vi "电压采样检测.vi"() -> ()   [LabVIEW 2020]
uses:
  D/Program Files (x86)/National Instruments/LabVIEW 2020/instr.lib/Keithley 24XX/Public/Data/Read (Single Point).vi
  D/Program Files (x86)/National Instruments/LabVIEW 2020/instr.lib/Keithley 24XX/Keithley 24XX.lvlib
panel:
  out "表格控件":string[][](table) caption="电压采样精度检测"
  out "?":bool
  out "电压 3":cluster{"Va":u32, "Vc":u32, "Vd":u32, "Vg":u32}
  out "闭合主正+快充":cluster{"Va":u32, "Vc":u32, "Vd":u32, "Vg":u32}
  in  "VISA resource name":refnum<visa-resource-name>
  out "闭合主正":cluster{"Va":u32, "Vc":u32, "Vd":u32, "Vg":u32}
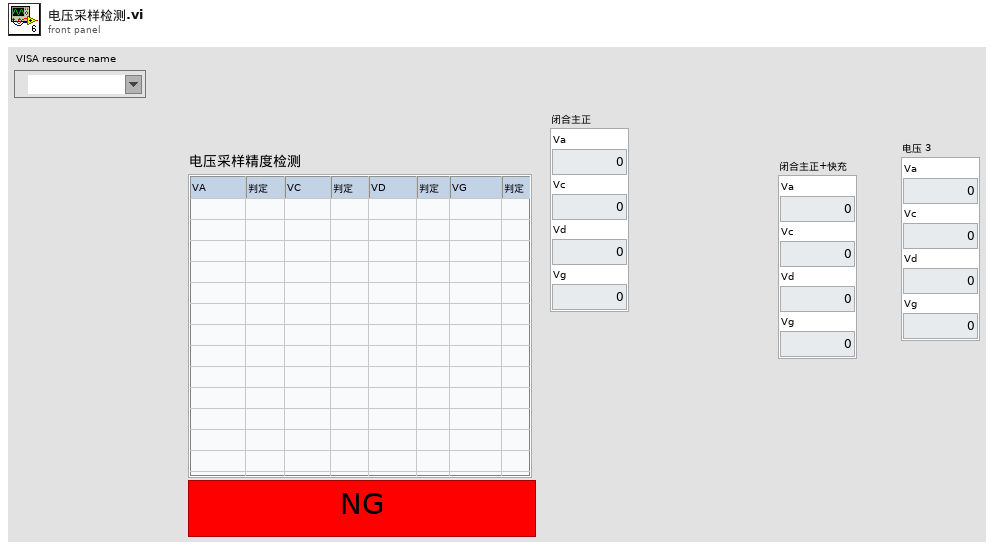
[diagram p1: front panel]
types:
  T1 = cluster{"电压[0]":u32, "电压[1]":u32, "电压[2]":u32, "电压[3]":u32}
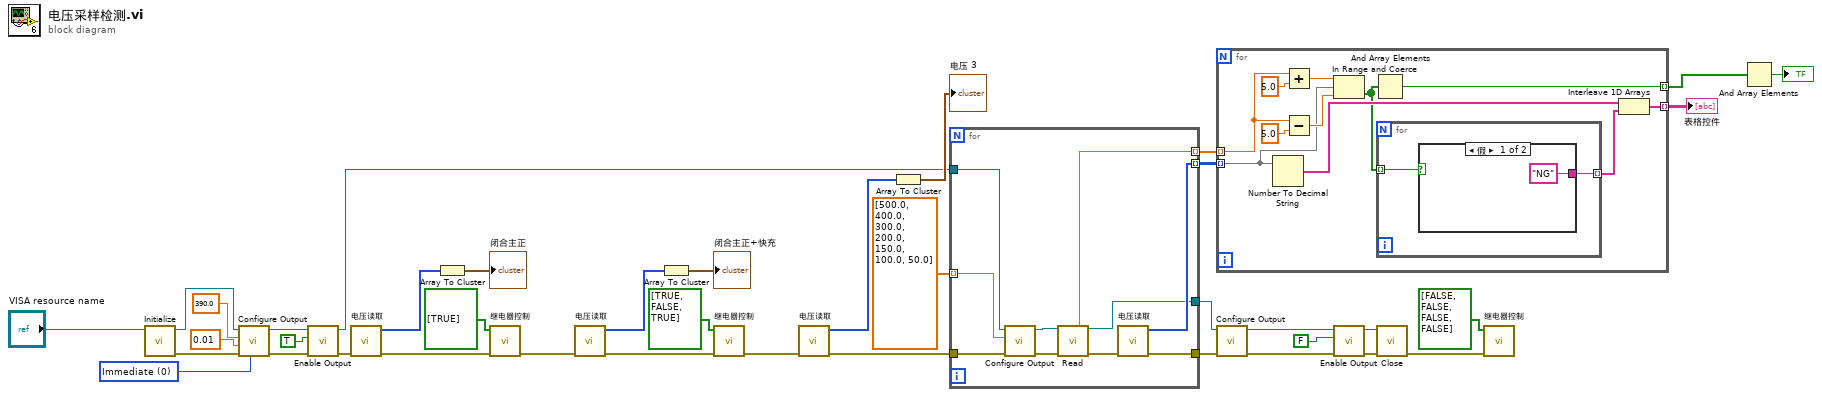
[diagram p0: block diagram]
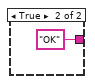
[diagram p2: hidden frame]
diagram:
  w32 = u16 0 items=["Immediate", "Triggered"] ("Output Type  (0: Immediate)")
  n1 = call "Initialize.vi"("VISA resource name"="VISA resource name") -> ("error out"=w33:errorcluster, "VISA resource name out"=w34:refnum<visa-resource-name>)  [unwired: 9 in]
  n2 = call "Configure Output.vi"("Output Type  (0: Immediate)"=w32, "error in (no error)"=w33, "Compliance  Level (0.1)"=0.01, "Output Level (0)"=390.0, "VISA resource name"=w34) -> ("error out"=w31:errorcluster, "VISA resource name out"=w30:refnum<visa-resource-name>)  [unwired: 5 in]
  n3 = call "Enable Output.vi"("error in (no error)"=w31, "Enable Output (T: Enable)"=TRUE, "VISA resource name"=w30) -> ("error out"=w28:errorcluster, "VISA resource name out"=w16:refnum<visa-resource-name>)  [unwired: 7 in]
  n4 = call "电压读取.vi"("error in"=w28) -> ("error out"=w27:errorcluster, "电压"=w39:u32[])  [unwired: 9 in]
  n5 = Array To Cluster(array=w39) -> (cluster=→"闭合主正":T1)
  n6 = call "继电器控制.vi"("error in"=w27, "继电器控制"=bool[] [TRUE]) -> ("error out"=w25:errorcluster)  [unwired: 9 in]
  n7 = call "电压读取.vi"("error in"=w25) -> ("error out"=w22:errorcluster, "电压"=w23:u32[])  [unwired: 9 in]
  n8 = Array To Cluster(array=w23) -> (cluster=→"闭合主正+快充":T1)
  n9 = call "继电器控制.vi"("error in"=w22, "继电器控制"=bool[] [TRUE, FALSE, TRUE]) -> ("error out"=w20:errorcluster)  [unwired: 9 in]
  n10 = call "电压读取.vi"("error in"=w20) -> ("error out"=w6:errorcluster, "电压"=w18:u32[])  [unwired: 9 in]
  n11 = Array To Cluster(array=w18) -> (cluster=→"电压 3":T1)
  n12 = for {
    tunnel: dbl[] [500.0, 400.0, 300.0, 200.0, 150.0, 100.0, 50.0] -> [w49] mode=indexing
    tunnel: w16 -> [w48]
    tunnel: [w47] -> w15
    tunnel: [w41] -> w14
    tunnel: [w46] -> w5 mode=indexing
    tunnel: w6 -> [w45]
    tunnel: [w40] -> w4 mode=indexing
    n13 = call "Configure Output.vi"("error in (no error)"=w45, "Output Level (0)"=w49, "VISA resource name"=w48) -> ("error out"=w44:errorcluster, "VISA resource name out"=w42:refnum<visa-resource-name>)  [unwired: 7 in]
    n14 = call-poly "Read.vi"("VISA resource name"=w42, "error in (no error)"=w44) -> ("Voltage"=w40:sgl, "VISA resource name out"=w41:refnum<visa-resource-name>, "error out"=w43:errorcluster)  [unwired: 7 in, 4 out]
    n15 = call "电压读取.vi"("error in"=w43) -> ("error out"=w47:errorcluster, "电压"=w46:u32[])  [unwired: 9 in]
  }
  n16 = for {
    tunnel: w5 -> [w55] mode=indexing
    tunnel: w4 -> [w58] mode=indexing
    tunnel: [w52] -> w1 mode=indexing
    tunnel: [w50] -> w3 mode=indexing
    n17 = Number To Decimal String(number=w55) -> (decimal integer string=w54:string[])  [unwired: 1 in]
    n18 = Add(x=w58, y=5.0) -> (x+y=w57:dbl)
    n19 = Subtract(x=w58, y=5.0) -> (x-y=w56:dbl)
    n20 = In Range and Coerce(upper limit=w57, x=w55, lower limit=w56) -> (In Range?=w51:bool[])  [unwired: 1 out]
    n21 = And Array Elements(Boolean array=w51) -> (logical AND=w50:bool)
    n22 = for {
      tunnel: w51 -> [w62] mode=indexing
      tunnel: [w61] -> w53 mode=indexing
      n23 = case shown="假" w62 {
        tunnel: ["NG" "OK"] -> w61
        frame False {
        }
        frame True {
        }
      }
    }
    n24 = Interleave 1D Arrays(w54, w53) -> (w52:string[])
  }
  "表格控件" <- w1
  n25 = call "Configure Output.vi"("error in (no error)"=w15, "VISA resource name"=w14) -> ("error out"=w13:errorcluster, "VISA resource name out"=w12:refnum<visa-resource-name>)  [unwired: 8 in]
  n26 = call "Enable Output.vi"("error in (no error)"=w13, "Enable Output (T: Enable)"=FALSE, "VISA resource name"=w12) -> ("error out"=w9:errorcluster, "VISA resource name out"=w7:refnum<visa-resource-name>)  [unwired: 7 in]
  n27 = call "Close.vi"("error in (no error)"=w9, "VISA resource name"=w7) -> ("error out"=w8:errorcluster)  [unwired: 9 in]
  n28 = call "继电器控制.vi"("error in"=w8, "继电器控制"=bool[] [FALSE, FALSE, FALSE, FALSE]) -> ()  [unwired: 9 in, 1 out]
  n29 = And Array Elements(Boolean array=w3) -> (logical AND=→"?":bool)
